vi "Read Local Dispatcher Port.vi"(11 "error in":errorcluster) -> (4 "UDP port":u16, 15 "error out":errorcluster)   [LabVIEW 2015, in "TLB` Template.lvlib" / "AMC.lvlib"]
doc: "Returns the UDP Port used by the local Dispatcher.TLB Prime - Application Template 1.3.0.24\nNorm Kirchner, NI Systems Engineering - NI\nCopyright (c) 2014, NI"
uses:
  AMC.lvlib
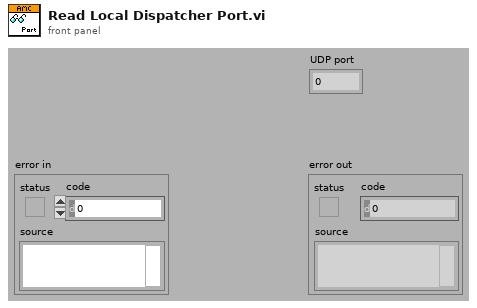
[diagram p1: front panel]
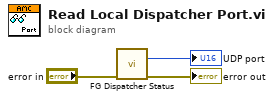
[diagram p0: block diagram]
diagram:
  n1 = call "FG Dispatcher Status.vi"("error in"="error in") -> ("UDP port out"=→"UDP port":u16, "error out"=→"error out":errorcluster)  [unwired: 12 in, 1 out]
